vi "FlashWindow.vi"(8 "No Error":errorcluster, 10 "Flash Operation":T1, 11 "Window [SDL_Window *]":T2 format="%.0x") -> (0 "Error Out":errorcluster)   [LabVIEW 2026, in "SDL3.lvlib" / "Video.lvlib"]
doc: "<B>Summary</B>\nRequest a window to demand attention from the user."
uses:
  Video.lvlib
  FlashOperation--enum.ctl
  <vilib>/Utility/error.llb/Error Cluster From Error Code.vi
  Error/Error.lvlib
  Lib/SDL3.dll
  SDL_Window--pointer.ctl
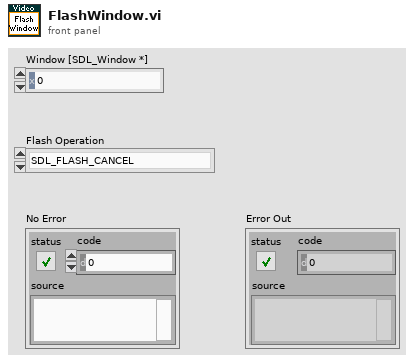
[diagram p1: front panel]
types:
  T1 = typedef "SDL3.lvlib/Video.lvlib/FlashOperation--enum.ctl" = enum32{"SDL_FLASH_CANCEL", "SDL_FLASH_BRIEFLY", "SDL_FLASH_UNTIL_FOCUSED"}
  T2 = typedef "SDL3.lvlib/Video.lvlib/SDL_Window--pointer.ctl" = i64
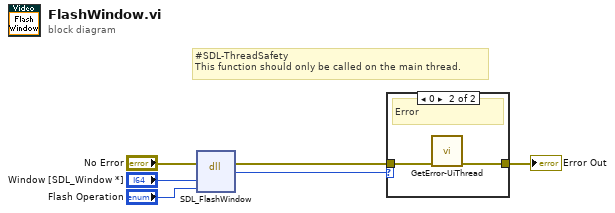
[diagram p0: block diagram]
diagram:
  # "#SDL-ThreadSafety\nThis function should only be called on the main thread."
  n1 = dll-call lib="C:/Users/saukko/Dev/LV-SDL3/Sources/SDL3/Lib/SDL3.*" fn="SDL_FlashWindow"(error in="No Error", "window"="Window [SDL_Window *]", "operation"="Flash Operation") -> (error out=w2:errorcluster, "return type"=w1:i32)  [unwired: 4 in, 1 out]
  n2 = case shown="0" w1 {
    tunnel: w2 -> [w7 w9]
    tunnel: [w7 w8] -> w5
    frame Default {
      # "Ok"
    }
    frame 0 {
      # "Error"
      n3 = call "GetError-UiThread.vi"("No Error"=w9) -> ("error out"=w8:errorcluster)  [unwired: 10 in]
    }
  }
  "Error Out" <- w5
